vi "SubVI_Example_MemoryAllocation.vi"(0 ".NET (Reference)":refnum<k24>, 5 "Error In":errorcluster) -> (14 "Bits/Pixel 2":i32=8, 15 "Width":i32, 16 "Serial Number":string, 17 "Height":i32, 19 "Error Out":errorcluster)   [LabVIEW 2017]
uses:
  C:/Users/George Sirinakis/Desktop/Microscope Control/Device Library/Cameras/IDS/IDS LabView Examples/LabVIEW/ueye.NET/uEyeDotNet.dll
  uEyeDotNet.dll
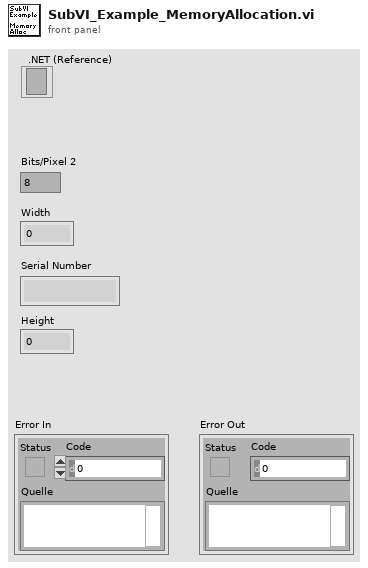
[diagram p1: front panel]
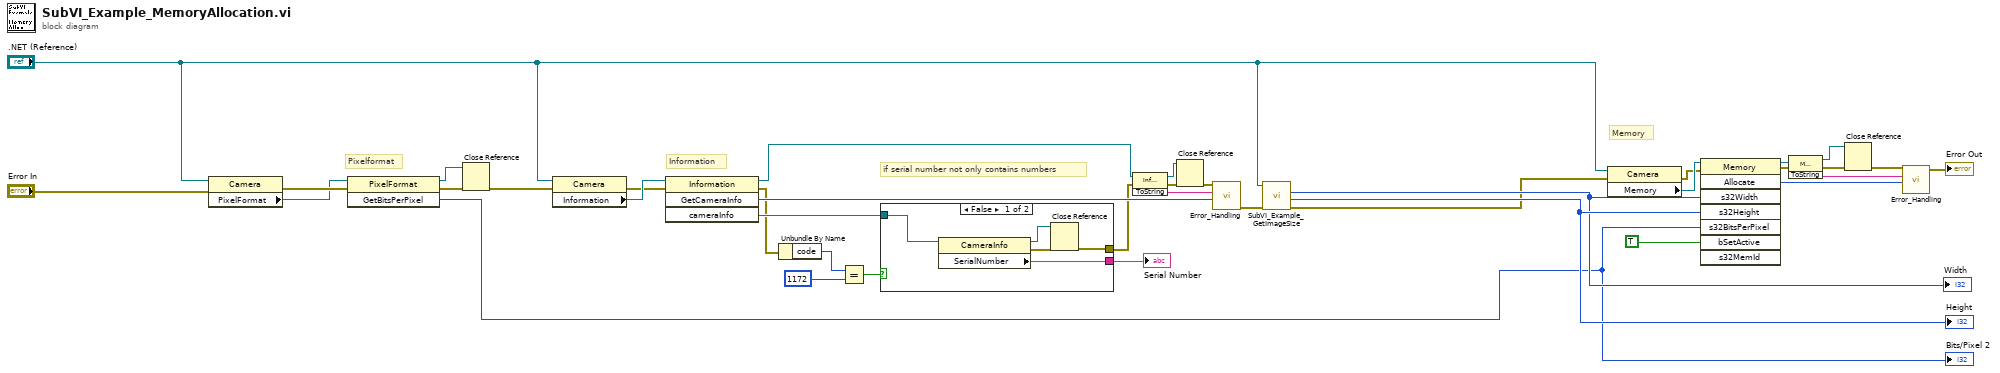
[diagram p0: block diagram]
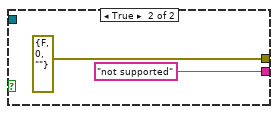
[diagram p2: hidden frame]
diagram:
  # "if serial number not only contains numbers"
  # "Information"
  # "Memory"
  # "Pixelformat"
  n1 = property class="Camera"(reference=".NET (Reference)", error in="Error In") -> (error out=w27:errorcluster, "PixelFormat"=w26:refnum<k24>)  [unwired: 1 out]
  n2 = invoke class="PixelFormat" method="GetBitsPerPixel"(reference=w26, error in=w27) -> (reference out=w9:refnum<k24>, error out=w11:errorcluster, "GetBitsPerPixel"=w12:i32)  [unwired: 1 in]
  "Bits/Pixel 2" <- w12
  n3 = Close Reference(reference=w9, error in (no error)=w11) -> (error out=w10:errorcluster)
  n4 = property class="Camera"(reference=".NET (Reference)", error in=w10) -> (error out=w24:errorcluster, "Information"=w25:refnum<k24>)  [unwired: 1 out]
  n5 = invoke class="Information" method="GetCameraInfo"(reference=w25, error in=w24) -> (reference out=w38:refnum<k24>, error out=w8:errorcluster, "GetCameraInfo"=w37:i32, "cameraInfo"=w19:refnum<k24>)  [unwired: 2 in]
  n6 = Unbundle By Name(w8) -> ("code"=w20:i32)
  n7 = Equal?(x=w20, y=1172) -> (x = y?=w22:bool)
  n8 = case shown="False" w22 {
    tunnel: [w40 errorcluster {"status"=FALSE, "code"=0, "source"=""} ("Error Out")] -> w17
    tunnel: w19 -> [w43 _]
    tunnel: [w42 "not supported"] -> w18
    frame False {
      n9 = property class="CameraInfo"(reference=w43) -> (reference out=w39:refnum<k24>, error out=w41:errorcluster, "SerialNumber"=w42:string)  [unwired: 1 in]
      n10 = Close Reference(reference=w39, error in (no error)=w41) -> (error out=w40:errorcluster)
    }
    frame True {
    }
  }
  "Serial Number" <- w18
  n11 = invoke class="Information" method="ToString"(reference=w38, error in=w17) -> (reference out=w5:refnum<k24>, error out=w7:errorcluster, "ToString"=w36:string)  [unwired: 1 in]
  n12 = Close Reference(reference=w5, error in (no error)=w7) -> (error out=w6:errorcluster)
  n13 = call "Error_Handling.vi"("Error Code"=w37, "Error String"=w36, "Error In"=w6) -> ("Error Out"=w16:errorcluster)  [unwired: 8 in]
  n14 = call "SubVI_Example_GetImageSize.vi"("Error In"=w16, ".NET (Reference)"=".NET (Reference)") -> ("Error Out"=w13:errorcluster, "Height"=w15:i32, "Width"=w14:i32)  [unwired: 6 in, 1 out]
  "Height" <- w15
  "Width" <- w14
  n15 = property class="Camera"(reference=".NET (Reference)", error in=w13) -> (error out=w28:errorcluster, "Memory"=w29:refnum<k24>)  [unwired: 1 out]
  n16 = invoke class="Memory" method="Allocate"(reference=w29, error in=w28, "s32Width"=w14, "s32Height"=w15, "s32BitsPerPixel"=w12, "bSetActive"=TRUE) -> (reference out=w34:refnum<k24>, error out=w33:errorcluster, "Allocate"=w32:i32)  [unwired: 2 in, 5 out]
  n17 = invoke class="Memory" method="ToString"(reference=w34, error in=w33) -> (reference out=w3:refnum<k24>, error out=w4:errorcluster, "ToString"=w31:string)  [unwired: 1 in]
  n18 = Close Reference(reference=w3, error in (no error)=w4) -> (error out=w2:errorcluster)
  n19 = call "Error_Handling.vi"("Error Code"=w32, "Error String"=w31, "Error In"=w2) -> ("Error Out"=→"Error Out":errorcluster)  [unwired: 8 in]
